vi "AlliGator Get Phasor Ratio Reference v2.vi"(8 "Error In":errorcluster, 9 "Last Phasor":T1, 11 "Data":variant) -> (0 "error out":errorcluster, 1 "Reference #":i32, 3 "Reference Phasor":T1)   [LabVIEW 2021, in "AlliGator Phasor Ratio.lvlib"]
doc: "Gets the phasor reference selected by the user."
uses:
  AlliGator Phasor Ratio.lvlib
  Phasor/Phasor (g, s).ctl
  AlliGator Phasor Reference Data.ctl
  Graphs/XY Graph/XY Graph Mouse Click Event Data.ctl
  Graphs/XY Graph/XY Graph Refnum.ctl
  <vilib>/Utility/miscctls.llb/LVPoint32TypeDef.ctl
  Graphs/XY Graph/XY Graph Add-Ons.lvlib
  Phasor/Phasor.lvlib
  AlliGator Phasor Plot.lvlib
panel:
  # "see the AlliGator License on the block diagram (Ctrl+E or Window:Show Block Diagram)"
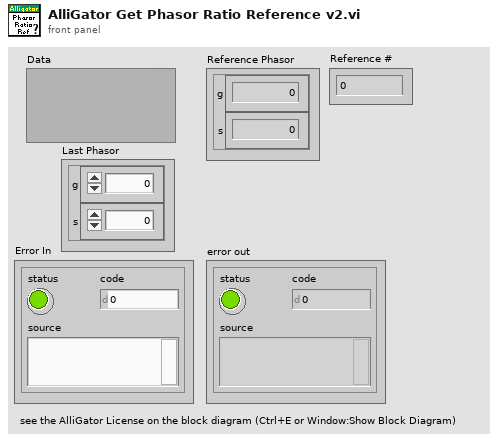
[diagram p1: front panel]
types:
  T1 = typedef "Phasor.lvlib/Phasor (g, s).ctl" = cluster{"g":dbl, "s":dbl}
  T2 = typedef "AlliGator Phasor Ratio.lvlib/AlliGator Phasor Reference Data.ctl" = cluster{"Data Type":string, "Data":variant}
  T3 = typedef "XY Graph Add-Ons.lvlib/XY Graph Mouse Click Event Data.ctl" = cluster{"Multiplot XY Graph":T4, "Mouse Coordinates":T5}
  T4 = typedef "XY Graph Add-Ons.lvlib/XY Graph Refnum.ctl" = refnum<vi>
  T5 = typedef "LVPoint32TypeDef.ctl" = cluster{"Horizontal":i32, "Vertical":i32}
  T6 = cluster{"Mouse Click Event Data":T3, "Reference #":i32}
  T7 = cluster{"Last Mouse Position":cluster{"X":i32, "Y":i32}, "Reference #":i32}
  T8 = typedef "AlliGator Phasor Plot.lvlib/AlliGator Phasor Plot Size.ctl" = cluster{"H":i32, "V":i32, "Margin":dbl}
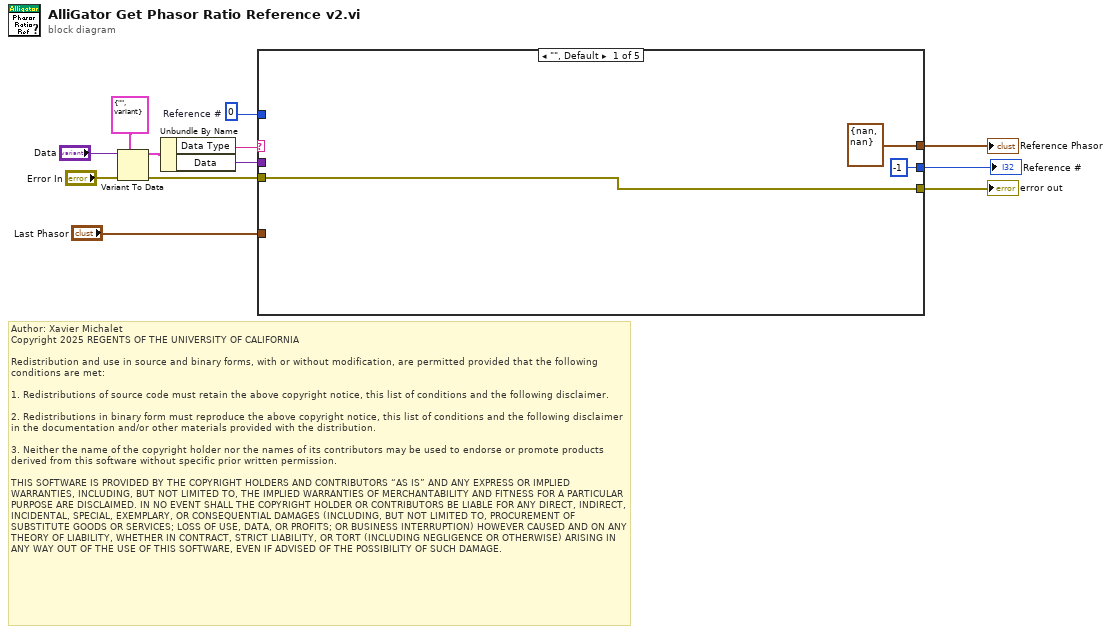
[diagram p0: block diagram]
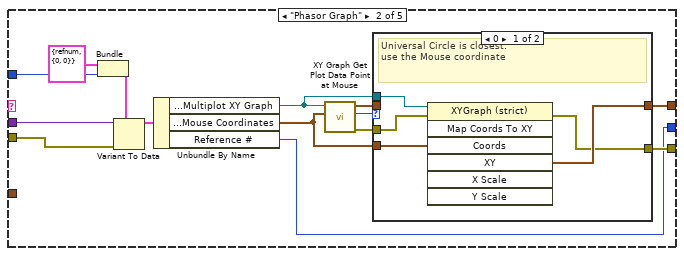
[diagram p2: hidden frame]
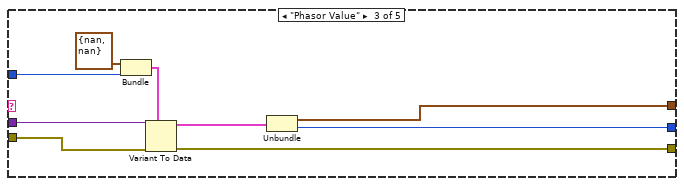
[diagram p4: hidden frame]
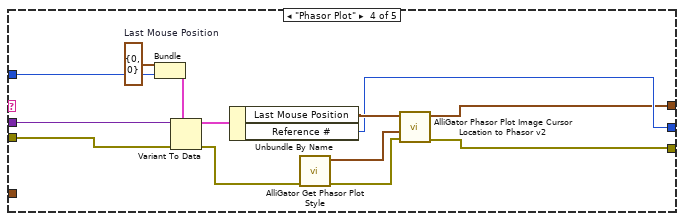
[diagram p5: hidden frame]
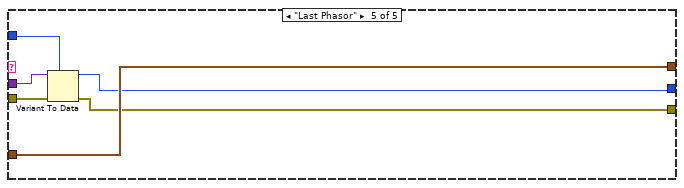
[diagram p6: hidden frame]
diagram:
  w5 = 0  # Reference #
  # "Author: Xavier Michalet\nCopyright 2025 REGENTS OF THE UNIVERSITY OF CALIFORNIA\n\nRedistribution and use in source and binary forms, with or without modification, are permitted provided that the following conditions are met:\n\n1. Redistributions of source code must retain the above copyright notice, this list of conditions and the following disclaimer.\n\n2. Redistributions in binary form must reproduce the above copyright notice, this list of conditions and the following disclaimer in the documentation and/or other materials provided with the distribution.\n\n3. Neither the name of the copyright holder nor the names of its contributors may be used to endorse or promote products derived from this software without specific prior written permission.\n\nTHIS SOFTWARE IS PROVIDED BY THE COPYRIGHT HOLDERS AND CONTRIBUTORS “AS IS” AND ANY EXPRESS OR IMPLIED WARRANTIES, INCLUDING, BUT NOT LIMITED TO, THE IMPLIED WARRANTIES OF MERCHANTABILITY AND FITNESS FOR A PARTICULAR PURPOSE ARE DISCLAIMED. IN NO EVENT SHALL THE COPYRIGHT HOLDER OR CONTRIBUTORS BE LIABLE FOR ANY DIRECT, INDIRECT, INCIDENTAL, SPECIAL, EXEMPLARY, OR CONSEQUENTIAL DAMAGES (INCLUDING, BUT NOT LIMITED TO, PROCUREMENT OF SUBSTITUTE GOODS OR SERVICES; LOSS OF USE, DATA, OR PROFITS; OR BUSINESS INTERRUPTION) HOWEVER CAUSED AND ON ANY THEORY OF LIABILITY, WHETHER IN CONTRACT, STRICT LIABILITY, OR TORT (INCLUDING NEGLIGENCE OR OTHERWISE) ARISING IN ANY WAY OUT OF THE USE OF THIS SOFTWARE, EVEN IF ADVISED OF THE POSSIBILITY OF SUCH DAMAGE."
  n1 = Variant To Data(error in="Error In", type=T2 {"Data Type"="", "Data"=variant} ("Phasor Reference Data"), Variant="Data") -> (data=w9:T2, error out=w6:errorcluster)
  n2 = Unbundle By Name(w9) -> ("Data Type"=w8:string, "Data"=w7:variant)
  n3 = case shown="\"\", Default" w8 {
    tunnel: w7 -> [_ w29 w43 w50 w63]
    tunnel: w6 -> [w15 w28 w41 w49 w62]
    tunnel: [T1 {"g"=nan, "s"=nan} ("Last Phasor") w19 w39 w47 w64] -> w1
    tunnel: [w15 w18 w37 w46 w59] -> w3
    tunnel: w5 -> [_ w17 w42 w51 w61]
    tunnel: [-1 ("Reference #") w16 w38 w48 w60] -> w2
    tunnel: "Last Phasor" -> [_ _ _ _ w64]
    frame "", Default {
    }
    frame "Phasor Graph" {
      n4 = Bundle("Mouse Click Event Data"=T3 {"Multiplot XY Graph"=refnum, "Mouse Coordinates"={"Horizontal"=0, "Vertical"=0}}, "Reference #"=w17) -> (w26:T6)  [unwired: 1 in]
      n5 = Variant To Data(error in=w28, type=w26, Variant=w29) -> (data=w25:T6)  [unwired: 1 out]
      n6 = Unbundle By Name(w25) -> ("Mouse Click Event Data.Multiplot XY Graph"=w22:T4, "Mouse Click Event Data.Mouse Coordinates"=w20:T5, "Reference #"=w16:i32)
      n7 = call "XY Graph Get Plot Data Point at Mouse.vi"("Coords"=w20, "XYGraph in"=w22) -> ("Error Out"=w21:errorcluster, "Plot Number"=w24:i32, "Plot Data Point"=w23:cluster{"X":dbl, "Y":dbl})  [unwired: 5 in, 2 out]
      n8 = case shown="0" w24 {
        tunnel: w23 -> [_ w36]
        tunnel: [w31 w36] -> w19
        tunnel: w22 -> [w34 _]
        tunnel: w21 -> [w33 w35]
        tunnel: w20 -> [w32 _]
        tunnel: [w30 w35] -> w18
        frame 0 {
          # "Universal Circle is closest:\nuse the Mouse coordinate"
          n9 = invoke class="XYGraph (strict)" method="Map Coords To XY"(reference=w34, error in=w33, "Coords"=w32) -> (error out=w30:errorcluster, "XY"=w31:cluster{"X":dbl, "Y":dbl})  [unwired: 4 in, 5 out]
        }
        frame 1, Default {
          # "Other plots"
        }
      }
    }
    frame "Phasor Value" {
      n10 = Bundle("Current Phasor"=T1 {"g"=nan, "s"=nan}, "Reference #"=w42) -> (w45:cluster{"Current Phasor":T1, "Reference #":i32})  [unwired: 1 in]
      n11 = Variant To Data(error in=w41, type=w45, Variant=w43) -> (data=w40:cluster{"Current Phasor":T1, "Reference #":i32}, error out=w37:errorcluster)
      n12 = Unbundle(w40) -> ("Current Phasor"=w39:T1, "Reference #"=w38:i32)
    }
    frame "Phasor Plot" {
      w56 = cluster{"X":i32, "Y":i32} {"X"=0, "Y"=0}  # Last Mouse Position
      n13 = Bundle("Last Mouse Position"=w56, "Reference #"=w51) -> (w53:T7)  [unwired: 1 in]
      n14 = Variant To Data(error in=w49, type=w53, Variant=w50) -> (data=w57:T7, error out=w54:errorcluster)
      n15 = Unbundle By Name(w57) -> ("Last Mouse Position"=w58:cluster{"X":i32, "Y":i32}, "Reference #"=w48:i32)
      n16 = call "AlliGator Get Phasor Plot Style.vi"("Error In"=w54) -> ("Error Out"=w55:errorcluster, "Phasor Plot Size"=w52:T8)  [unwired: 8 in, 1 out]
      n17 = call "AlliGator Phasor Plot Image Cursor Location to Phasor v2.vi"("Error In"=w55, "Phasor Plot Size"=w52, "Coords in"=w58) -> ("Error Out"=w46:errorcluster, "Phasor"=w47:T1)  [unwired: 7 in]
    }
    frame "Last Phasor" {
      n18 = Variant To Data(error in=w62, type=w61, Variant=w63) -> (data=w60:i32, error out=w59:errorcluster)
    }
  }
  "Reference Phasor" <- w1
  "error out" <- w3
  "Reference #" <- w2
